vi "SENS_IF_FREQ_AUTO.vi"(0 "VISA IN":refnum<visa-resource-name>, 1 "AUTO ON/OFF":bool, 5 "error in":errorcluster, 7 "Channel":i32) -> (14 "VISA Out":refnum<visa-resource-name>, 19 "error out":errorcluster)   [LabVIEW 2018, in "PNA-X.lvlib"]
doc: "SENSe<cnum>:IF:FREQuency:AUTO <bool> \n1759\n\n(Read-Write) Sets and returns the method for specifying the way the IF Frequency is determined. \nCritical Note \nParameters \n<cnum> Existing channel number. If unspecified, <cnum> is set to 1. \n<bool> (Boolean) \nON (or 1) - Automatic. PNA determines the setting for the IF frequency. \nOFF (or 0) - Manual. Use SENS:IF:FREQ to set the frequency. \nExamples SENS:IF:FREQ:AUTO 1 \nsense2:if:frequency:auto 0 \nQuery Syntax SENSe<cnum>:IF:FREQuency:AUTO? \nReturn Type Boolean \nDefault ON"
uses:
  PNA-X.lvlib
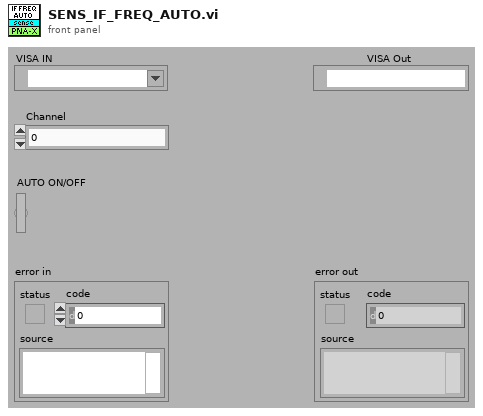
[diagram p1: front panel]
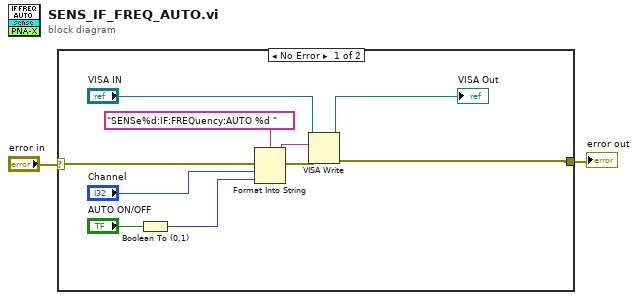
[diagram p0: block diagram]
diagram:
  n1 = case shown="No Error" "error in" {
    selector: "error in" -> [w12 w13]
    tunnel: [w7 w13] -> w1
    frame No Error {
      n2 = Boolean To (0,1)(Boolean="AUTO ON/OFF") -> (0, 1=w3:i16)
      n3 = Format Into String(format string="SENSe%d:IF:FREQuency:AUTO %d " ("Cmdline"), error in=w12, "Channel", w3) -> (resulting string=w10:string, error out=w11:errorcluster)  [unwired: 1 in]
      n4 = VISA Write(VISA resource name="VISA IN", write buffer=w10, error in (no error)=w11) -> (VISA resource name out=→"VISA Out":refnum<visa-resource-name>, error out=w7:errorcluster)  [unwired: 1 out]
    }
    frame Error {
    }
  }
  "error out" <- w1
